vi "Create Frame Pattern Script.vi"(8 "error in (no error)":errorcluster, 9 "ChipID":u8, 10 "Frame_Data":T1={"Pattern_Name"="", "Operation Mode"=enum."Normal", "BurstLength"=enum."0", "FSN"=0, "Start_Addr"=0, "Data"=[], "R/W?"=enum."Read", "Opcode"=[], "ChipID"=1, "num of wait cycle of read"=0} {"Data" format="%x"; "Start_Addr" format="%x"}, 11 "BML_Frame_SetID in":refnum<class "BML_Frame_SetID.lvclass">) -> (0 "error out":errorcluster, 3 "BML_Frame_SetID out":refnum<class "BML_Frame_SetID.lvclass">)   [LabVIEW 2018, in "BML_Frame_SetID.lvclass"]
uses:
  BML_Frame_SetID.lvclass
  C:/P4 Workspace/PC Client/Solutions/5g_eap/HiSi/trunk/1.0/BML_Pattern_Gen_Refactor/Classes/BML_Frame_Root/BML_Frame_Root.lvclass
  Config_Read/Frame_Data.ctl
  Config_Read/OperationMode.ctl
  Config_Read/BurstLength.ctl
  Config_Read/RW_Option.ctl
  BML_Frame_Root/Special Frame.ctl
  BML_Frame_SetID.lvclass/BML_Frame_SetID.ctl
  BML_Frame_Root/BML_Frame_Root.lvclass/BML_Frame_Root.ctl
  BML_Frame_Cmd/BML_Frame_Command.lvclass
  Config_Read/Config_Read_BML.lvclass
  BML_Frame_Root/BML_Frame_Root.lvclass
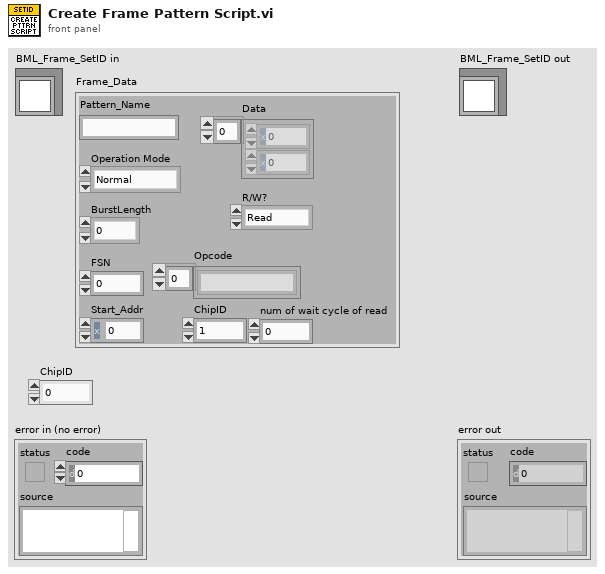
[diagram p1: front panel]
types:
  T1 = typedef "Config_Read_BML.lvclass/Frame_Data.ctl" = cluster{"Pattern_Name":string, "Operation Mode":T2, "BurstLength":T3, "FSN":u8, "Start_Addr":u16, "Data":u8[], "R/W?":T4, "Opcode":string[], "ChipID":u8, "num of wait cycle of read":i8}
  T2 = typedef "Config_Read_BML.lvclass/OperationMode.ctl" = enum8{"Normal", "ImmeEffect", "InitSlaveID", "LoadData"}
  T3 = typedef "Config_Read_BML.lvclass/BurstLength.ctl" = enum8{"0", "2", "3", "4", "5", "8", "16", "32"}
  T4 = typedef "Config_Read_BML.lvclass/RW_Option.ctl" = enum16{"Read", "Write", "R/W"}
  T5 = typedef "BML_Frame_Root.lvclass/Special Frame.ctl" = enum16{"Sync Header", "Protocol Header", "SW Trig", "SetID State", "Out SetID State", "SW Reset", "Wait", "SPI 4W FRM Start", "SPI 4W Wait", "SPI 4W FRM End", "SPI 4W Write Cmd", "SPI RD Collect Cmd", "SPI RD Value Cmd", "SPI 3W FRM Start", "SPI 3W Write Cmd", "SPI 3W FRM End", "SPI 3W Wait", "SPI 3W RD Cmd"}
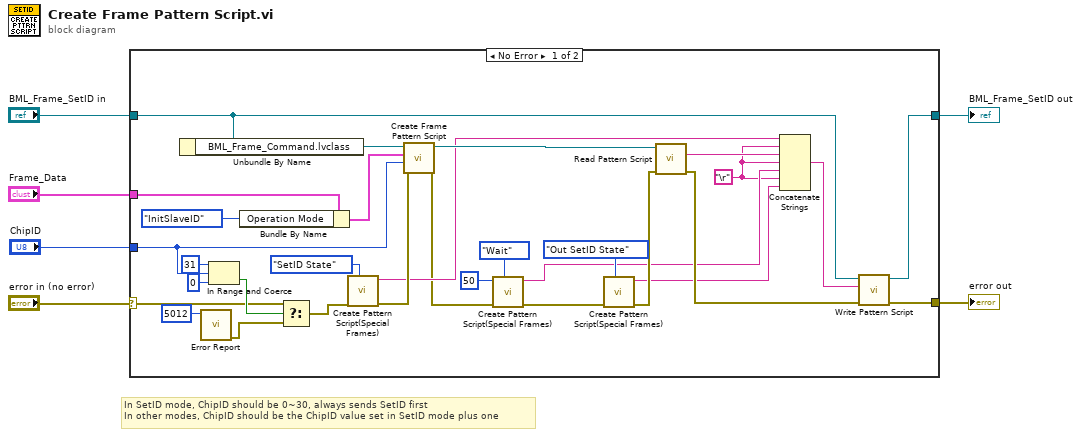
[diagram p0: block diagram]
diagram:
  # "In SetID mode, ChipID should be 0~30, always sends SetID first\nIn other modes, ChipID should be the ChipID value set in SetID mode plus one"
  n1 = case shown="No Error" "error in (no error)" {
    selector: "error in (no error)" -> [w10 w38]
    tunnel: "BML_Frame_SetID in" -> [w24 w39]
    tunnel: "Frame_Data" -> [w36 _]
    tunnel: "ChipID" -> [w14 _]
    tunnel: [w23 w39] -> w2
    tunnel: [w22 w38] -> w1
    frame No Error {
      w17 = "\r"
      n2 = Unbundle By Name(w24) -> ("BML_Frame_Command.lvclass"=w37:refnum<class "BML_Frame_Command.lvclass">)
      n3 = call "Error Report.vi"("Error Code"=i16 5012) -> ("error out"=w8:errorcluster)  [unwired: 10 in]
      n4 = In Range and Coerce(upper limit=u8 31, x=w14, lower limit=u8 0) -> (In Range?=w11:bool)  [unwired: 1 out]
      n5 = Bundle By Name(cluster=w36, "Operation Mode"=OperationMode."InitSlaveID") -> (w34:T1)
      n6 = Select(t=w10, s=w11, f=w8) -> (s? t:f=w9:errorcluster)
      n7 = call "Create Pattern Script(Special Frames).vi"("Special Frame Type"=Special_Frame."SetID State", "error in (no error)"=w9) -> ("error out"=w30:errorcluster, "string out"=w29:string)  [unwired: 8 in]
      n8 = call-dynamic "Create Frame Pattern Script.vi"("error in (no error)"=w30, "ChipID"=w14, "Frame_Data"=w34, "BML_Frame_Command in"=w37) -> ("error out"=w21:errorcluster, "BML_Frame_Command out"=w32:refnum<class "BML_Frame_Command.lvclass">)  [unwired: 6 in]
      n9 = call "Create Pattern Script(Special Frames).vi"("Special Frame Type"=Special_Frame."Wait", "error in (no error)"=w21, "Num of Timeset"=u32 50) -> ("error out"=w20:errorcluster, "string out"=w18:string)  [unwired: 7 in]
      n10 = call "Create Pattern Script(Special Frames).vi"("Special Frame Type"=Special_Frame."Out SetID State", "error in (no error)"=w20) -> ("error out"=w27:errorcluster, "string out"=w15:string)  [unwired: 8 in]
      n11 = call "Read Pattern Script.vi"("error in (no error)"=w27, "BML_Frame_Root in"=w32) -> ("error out"=w26:errorcluster, "Pattern Script"=w31:string)  [unwired: 7 in, 1 out]
      n12 = Concatenate Strings(w29, w17, w31, w17, w18, w17, w15) -> (w25:string)
      n13 = call "Write Pattern Script.vi"("error in (no error)"=w26, "Pattern Script"=w25, "BML_Frame_Root in"=w24) -> ("error out"=w22:errorcluster, "BML_Frame_Root out"=w23:refnum<class "BML_Frame_SetID.lvclass">)  [unwired: 7 in]
    }
    frame Error {
    }
  }
  "error out" <- w1
  "BML_Frame_SetID out" <- w2
